vi "Write SubPanel Ref.vi"(8 "error in (no error)":errorcluster, 10 "SubPanel Ref":refnum<vi>, 11 "Display Panel V3 in":refnum<class "Display Panel V3.lvclass">) -> (0 "error out":errorcluster, 3 "Display Panel V3 out":refnum<class "Display Panel V3.lvclass">)   [LabVIEW 2014]
uses:
  Display Panel V3.lvclass
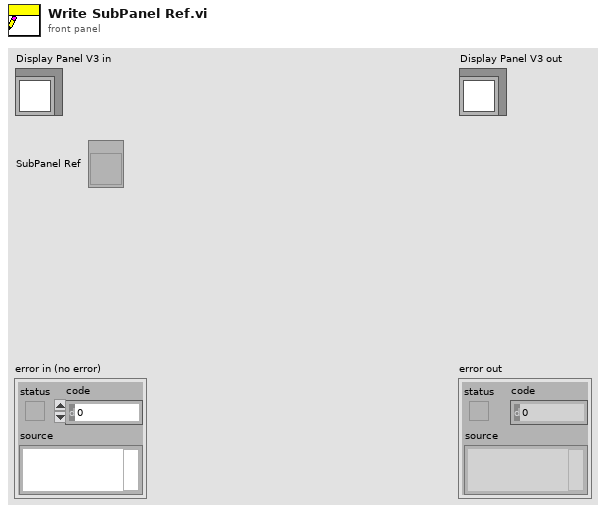
[diagram p1: front panel]
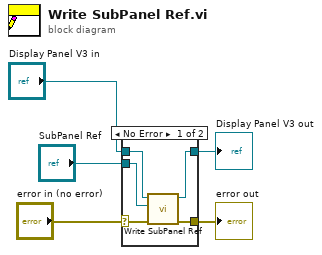
[diagram p0: block diagram]
diagram:
  n1 = case shown="No Error" "error in (no error)" {
    selector: "error in (no error)" -> [w7 w11]
    tunnel: [w6 w11] -> w4
    tunnel: [w9 w12] -> w2
    tunnel: "Display Panel V3 in" -> [w10 w12]
    tunnel: "SubPanel Ref" -> [w8 _]
    frame No Error {
      n2 = call-dynamic "Write SubPanel Ref.vi"("error in (no error)"=w7, "SubPanel Ref"=w8, "Subpanel Inserter in"=w10) -> ("error out"=w6:errorcluster, "Subpanel Inserter out"=w9:refnum<class "Display Panel V3.lvclass">)  [unwired: 7 in]
    }
    frame Error {
    }
  }
  "error out" <- w4
  "Display Panel V3 out" <- w2
